vi "Init.vi"(0 "ClassReaderGOOP300 in":refnum<class "ClassReaderGOOP400.lvclass">, 1 "LvClassRef":refnum<vi>, 5 "error in (no error)":errorcluster) -> (14 "ClassReaderGOOP300 out":refnum<class "ClassReaderGOOP400.lvclass">, 19 "error out":errorcluster)   [LabVIEW 2020, in "ClassReaderGOOP400.lvclass"]
uses:
  ClassReaderGOOP400.lvclass
  Provider_EndevoGOOP300/ClassReaderGOOP300_class/ClassReaderGOOP300.lvclass
  ClassReaderGOOP400.lvclass/ClassReaderGOOP400.ctl
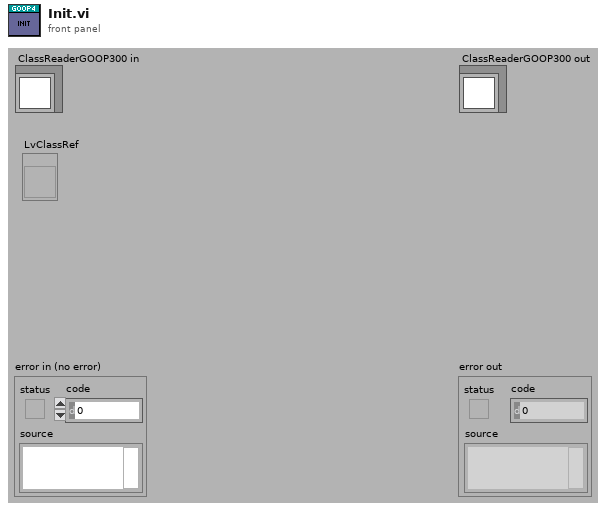
[diagram p1: front panel]
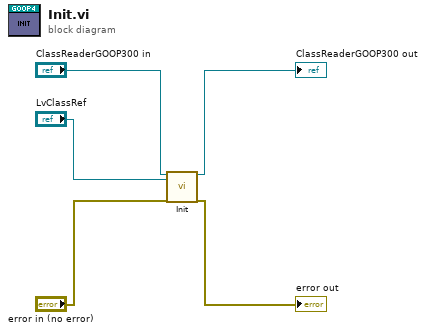
[diagram p0: block diagram]
diagram:
  n1 = call-parent "Init.vi"("ClassReaderGOOP300 in"="ClassReaderGOOP300 in", "LvClassRef"="LvClassRef", "error in (no error)"="error in (no error)") -> ("ClassReaderGOOP300 out"=→"ClassReaderGOOP300 out":refnum<class "ClassReaderGOOP400.lvclass">, "error out"=→"error out":errorcluster)  [unwired: 15 in]
